vi "Write Id.vi"(8 "error in (no error)":errorcluster, 10 "Id":string, 11 "CommandDirector in":refnum<class "CommandDirector.lvclass">) -> (0 "error out":errorcluster, 3 "CommandDirector out":refnum<class "CommandDirector.lvclass">)   [LabVIEW 2023, in "HAF.lvlib" / "CommandDirector.lvclass"]
doc: "Sets a new ID for this Director."
uses:
  CommandDirector.lvclass
  CommandDirector.lvclass/CommandDirector.ctl
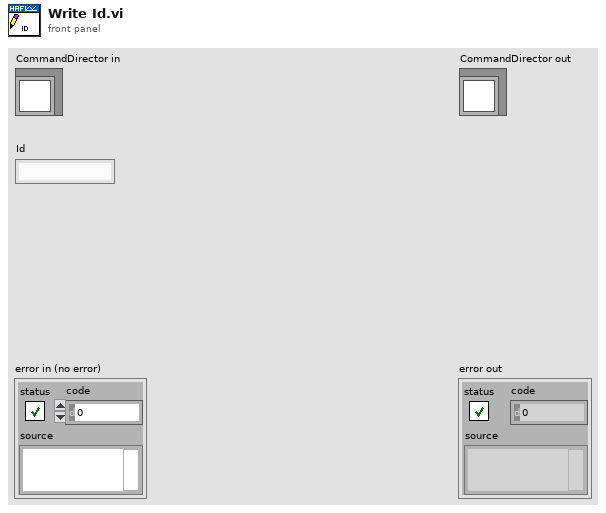
[diagram p1: front panel]
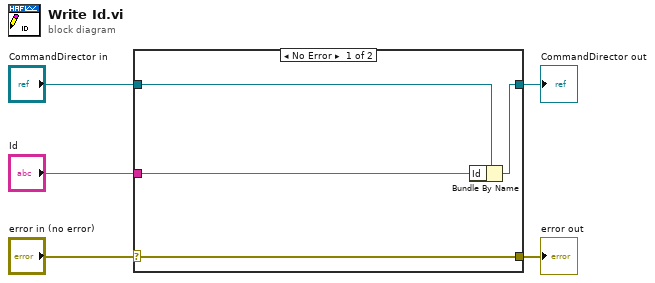
[diagram p0: block diagram]
diagram:
  n1 = case shown="No Error" "error in (no error)" {
    selector: "error in (no error)" -> [w9 w10]
    tunnel: [w9 w10] -> w4
    tunnel: [w7 w11] -> w2
    tunnel: "CommandDirector in" -> [w8 w11]
    tunnel: "Id" -> [w6 _]
    frame No Error {
      n2 = Bundle By Name(cluster=w8, "Id"=w6) -> (w7:refnum<class "CommandDirector.lvclass">)
    }
    frame Error {
    }
  }
  "error out" <- w4
  "CommandDirector out" <- w2
